vi "BRig_Host__Loop_Consumer_RunState__closedLoop_checkUpdateTrial.vi"(6 "input_forceUpdate":bool, 7 "input_nTrial":i32, 9 "input_updateID":u16, 10 "input_updateTrial_subsequent":u16, 11 "input_updateTrial_first":u16) -> (3 "output_update":bool)   [LabVIEW 2014]
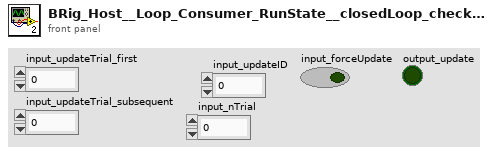
[diagram p1: front panel]
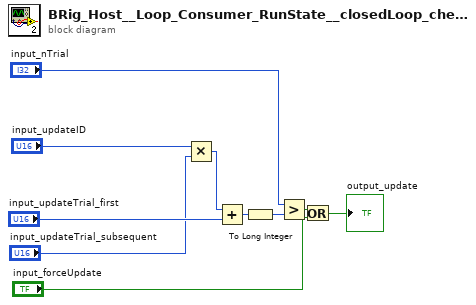
[diagram p0: block diagram]
diagram:
  n1 = Multiply(x="input_updateID", y="input_updateTrial_subsequent") -> (x*y=w7:u16)
  n2 = Add(x=w7, y="input_updateTrial_first") -> (x+y=w6:u16)
  n3 = To Long Integer(number=w6) -> (32bit integer=w4:i32)
  n4 = Greater?(x="input_nTrial", y=w4) -> (0:w5:bool)
  n5 = Or(x=w5, y="input_forceUpdate") -> (x .or. y?=→"output_update":bool)
